vi "Calculatrice 1.vi"() -> ()   [LabVIEW 2014]
panel:
  in  "stop":bool
  out "moy":dbl
  out "div":dbl
  out "mult":dbl
  out "sous":dbl
  out "add":dbl
  in  "Nmber1 2":dbl
  in  "Nmber1":dbl
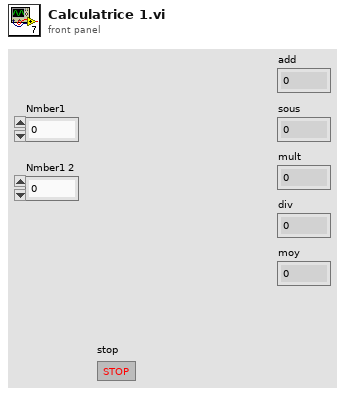
[diagram p1: front panel]
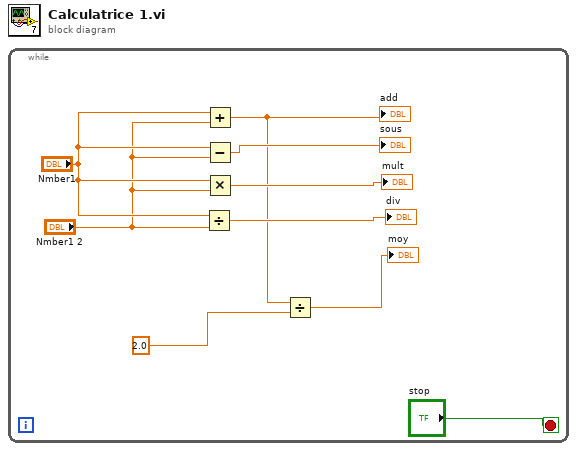
[diagram p0: block diagram]
diagram:
  n1 = while {
    stop <- "stop" stop-if-true
    n2 = Divide(x="Nmber1", y="Nmber1 2") -> (x/y=→"div":dbl)
    n3 = Add(x="Nmber1", y="Nmber1 2") -> (x+y=w5:dbl)
    "add" <- w5
    n4 = Subtract(x="Nmber1", y="Nmber1 2") -> (x-y=→"sous":dbl)
    n5 = Multiply(x="Nmber1", y="Nmber1 2") -> (x*y=→"mult":dbl)
    n6 = Divide(x=w5, y=2.0) -> (x/y=→"moy":dbl)
  }
